vi "QBPN-Create (AdvFilt).vi"(0 "Filter":T1 {"Stages"."IIR Filter"."Forward Coefficients" format="%.4f"; "Stages"."IIR Filter"."Reverse Coefficients" format="%.4f"}, 7 "Npts":i32=128, 11 "Omega (t)":dbl[](array[numeric])) -> (4 "Filter (out)":T1 {"Stages"."IIR Filter"."Forward Coefficients" format="%.4f"; "Stages"."IIR Filter"."Reverse Coefficients" format="%.4f"}, 8 "BP noise":dbl[](array[numeric]))   [LabVIEW 2020]
doc: "Create a token of bandpass noise using the quadrature filter method."
uses:
  Controls/Advanced Filter XCtl/Filter Data.ctl
  Filter VIs/Filter-Bandwidth Units.ctl
  <vilib>/Analysis/3filter.llb/IIR Cascade Filter with I.C. (DBL).vi
  <vilib>/Analysis/NI_AALBase.lvlib
  Controls/Advanced Filter XCtl/Advanced Filter XCtl.xctl
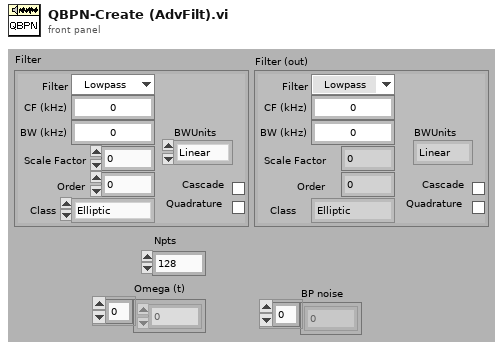
[diagram p1: front panel]
types:
  T1 = typedef "Advanced Filter XCtl.xctl/Filter Data.ctl" = cluster{"Type":enum16{"Lowpass", "Highpass", "Bandpass", "Bandstop", "OFF"}, "CF (kHz)":dbl, "BW (kHz)":dbl, "Cascade":bool, "Quadrature":bool, "Scale Factor":dbl, "Stages":cluster{"IIR Filter":cluster{"filter structure":enum32{"IIR 2nd Order", "IIR 4th Order"}, "Reverse Coefficients":dbl[], "Forward Coefficients":dbl[]}, "State":dbl[]}[], "Class":enum16{"Elliptic", "Butterworth"}, "Order":i32, "BWUnits":T2}
  T2 = typedef "Filter-Bandwidth Units.ctl" = enum16{"Linear", "Octaves", "Min-Max"}
  T3 = cluster{"IIR Filter":cluster{"filter structure":enum32{"IIR 2nd Order", "IIR 4th Order"}, "Reverse Coefficients":dbl[], "Forward Coefficients":dbl[]}, "State":dbl[]}[]
  T4 = cluster{"IIR Filter":cluster{"filter structure":enum32{"IIR 2nd Order", "IIR 4th Order"}, "Reverse Coefficients":dbl[], "Forward Coefficients":dbl[]}, "State":dbl[]}
  T5 = cluster{"filter structure":enum32{"IIR 2nd Order", "IIR 4th Order"}, "Reverse Coefficients":dbl[], "Forward Coefficients":dbl[]}
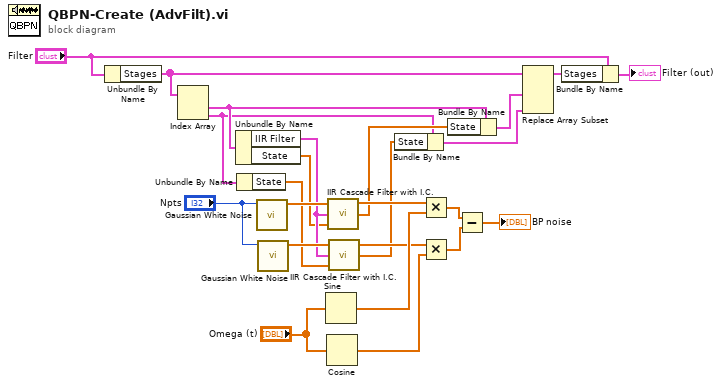
[diagram p0: block diagram]
diagram:
  n1 = Unbundle By Name("Filter") -> ("Stages"=w6:T3)
  n2 = Index Array(array=w6) -> (element #1=w10:T4, element #2=w8:T4)  [unwired: 2 in]
  n3 = Unbundle By Name(w10) -> ("IIR Filter"=w13:T5, "State"=w12:dbl[])
  n4 = Unbundle By Name(w8) -> ("State"=w11:dbl[])
  n5 = call <vilib>:"Gaussian White Noise.vi"("samples"="Npts") -> ("Gaussian noise pattern"=w23:dbl[])  [unwired: 9 in, 1 out]
  n6 = call <vilib>:"Gaussian White Noise.vi"("samples"="Npts") -> ("Gaussian noise pattern"=w24:dbl[])  [unwired: 9 in, 1 out]
  n7 = Sine(x="Omega (t)") -> (sin(x)=w22:dbl[])
  n8 = Cosine(x="Omega (t)") -> (cos(x)=w20:dbl[])
  n9 = call-poly <vilib>:"IIR Cascade Filter with I.C..vi"("Initial Filter State"=w12, "IIR Filter Cluster"=w13, "X"=w23) -> ("Final Filter State"=w9:dbl[], "Filtered X"=w17:dbl[])  [unwired: 1 out]
  n10 = call-poly <vilib>:"IIR Cascade Filter with I.C..vi"("Initial Filter State"=w11, "IIR Filter Cluster"=w13, "X"=w24) -> ("Final Filter State"=w7:dbl[], "Filtered X"=w21:dbl[])  [unwired: 1 out]
  n11 = Bundle By Name(cluster=w8, "State"=w7) -> (w4:T4)
  n12 = Multiply(x=w17, y=w22) -> (x*y=w19:dbl[])
  n13 = Multiply(x=w21, y=w20) -> (x*y=w18:dbl[])
  n14 = Bundle By Name(cluster=w10, "State"=w9) -> (w5:T4)
  n15 = Subtract(x=w19, y=w18) -> (x-y=→"BP noise":dbl[])
  n16 = Replace Array Subset(array=w6, new element #1=w5, new element #2=w4) -> (w2:T3)  [unwired: 2 in]
  n17 = Bundle By Name(cluster="Filter", "Stages"=w2) -> (→"Filter (out)":T1)
